vi "LVClass_Camera get all camera parameter values.vi"(0 "Camera in":refnum<class "Camera.lvclass">, 11 "error in (no error)":errorcluster) -> (4 "Camera out":refnum<class "Camera.lvclass">, 6 "ListOfSettableAndGettableValue":T1[](array[typedef]), 8 "nb_image":u32, 10 "BG Image OUT":refnum<class "Image.lvclass">, 15 "error out":errorcluster)   [LabVIEW 2020, in "Camera.lvclass"]
uses:
  Camera.lvclass
  Controls/CameraParametersSetup.ctl
  Controls/CameraParameters_Type.ctl
  Image/Image.lvclass
  Camera.lvclass/Camera.ctl
  LVClass_Camera Read acquisition state.vi
  LVClass_Camera Read all camera parameters.vi
  Image/LVClass_Image read Image Compat ptr.vi
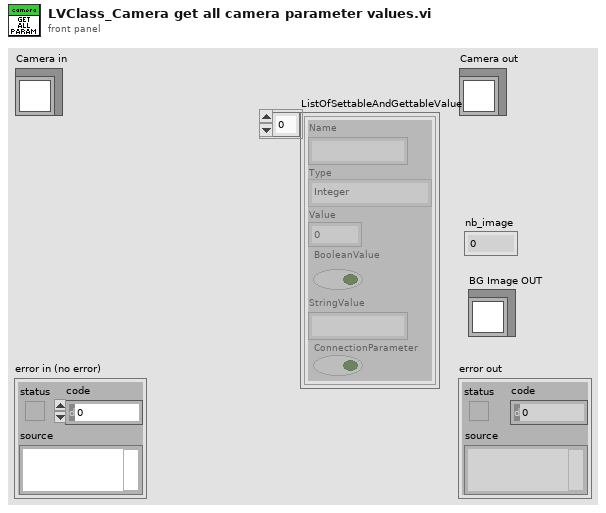
[diagram p1: front panel]
types:
  T1 = typedef "CameraParametersSetup.ctl" = cluster{"Name":string, "Type":T2, "Value":dbl, "BooleanValue":bool, "StringValue":string, "ConnectionParameter":bool}
  T2 = typedef "CameraParameters_Type.ctl" = enum16{"Integer", "Real", "String", "Boolean"}
  T3 = typedef "CameraAcquisitionState.ctl" = enum16{"Stop", "Live"}
  T4 = typedef "ParameterID.ctl" = cluster{"Name":string, "ConnectionParameter?":bool, "Type":T2, "Authorization":T5, "OnFlyAuthorization":T6, "StringValue":string, "Value":dbl, "Min":dbl, "Max":dbl, "BooleanValue":bool, "StringParameterList":string[]}
  T5 = typedef "CameraParameters_Authorization.ctl" = enum16{"Disable", "Gettable", "Settable - Gettable"}
  T6 = typedef "CameraParameters_OnFlyAuthorization.ctl" = enum16{"None", "Gettable", "Settable", "Settable - Gettable"}
  T7 = enum32{"invalid app kind", "Development System", "Run Time System", "Student Edition", "Embedded LabVIEW", "Evaluation", "Custom"}
  T8 = typedef "ClassID.ctl" = i64
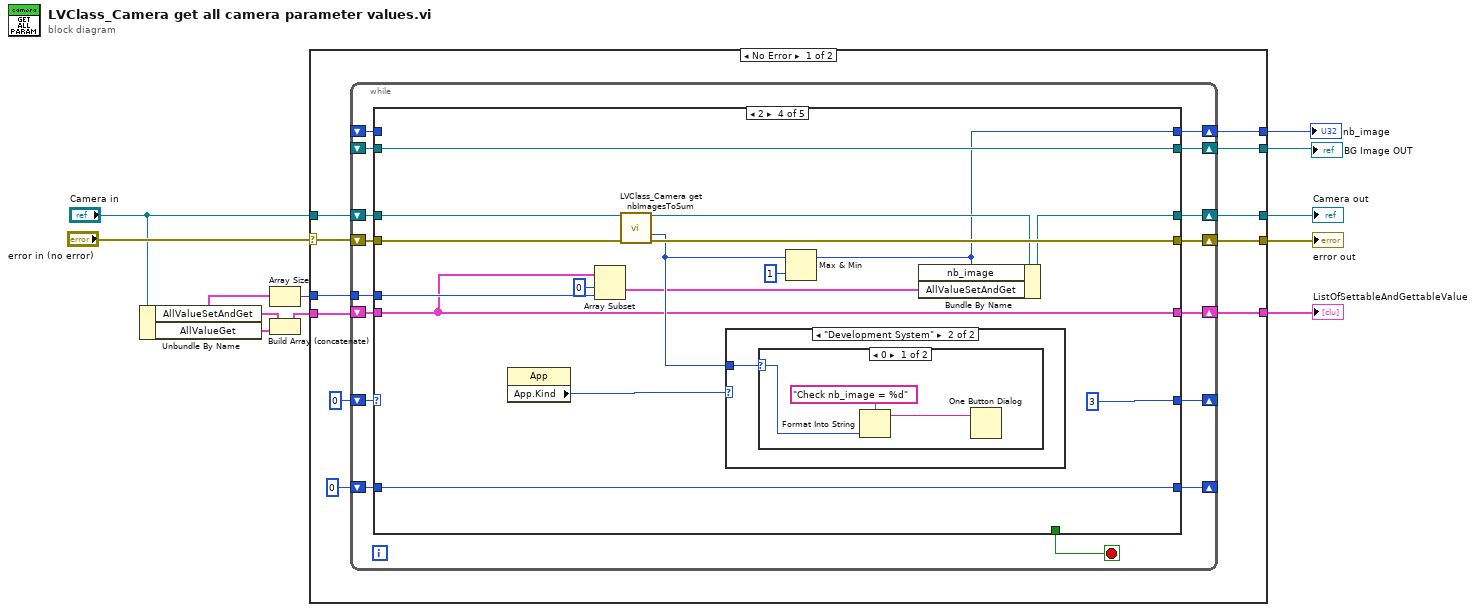
[diagram p0: block diagram]
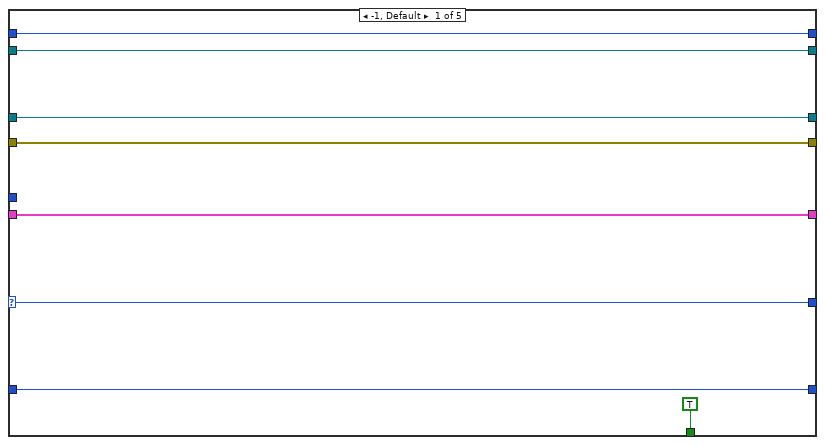
[diagram p2: hidden frame]
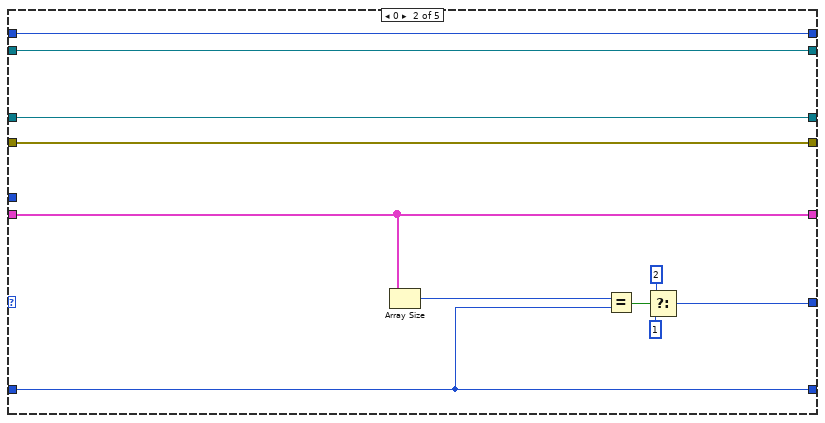
[diagram p3: hidden frame]
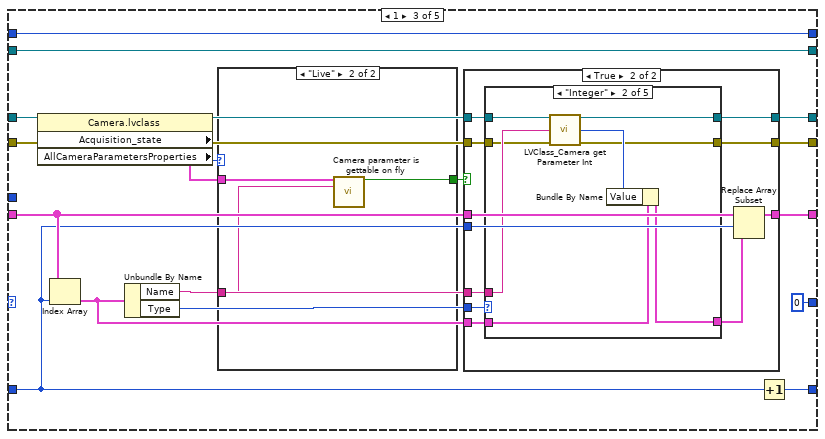
[diagram p4: hidden frame]
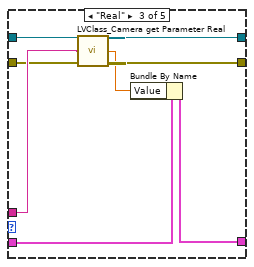
[diagram p7: hidden frame]
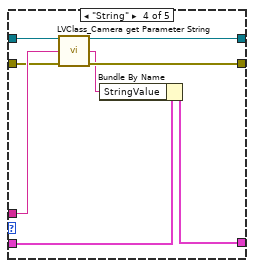
[diagram p8: hidden frame]
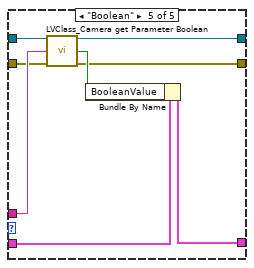
[diagram p9: hidden frame]
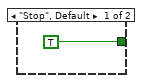
[diagram p10: hidden frame]
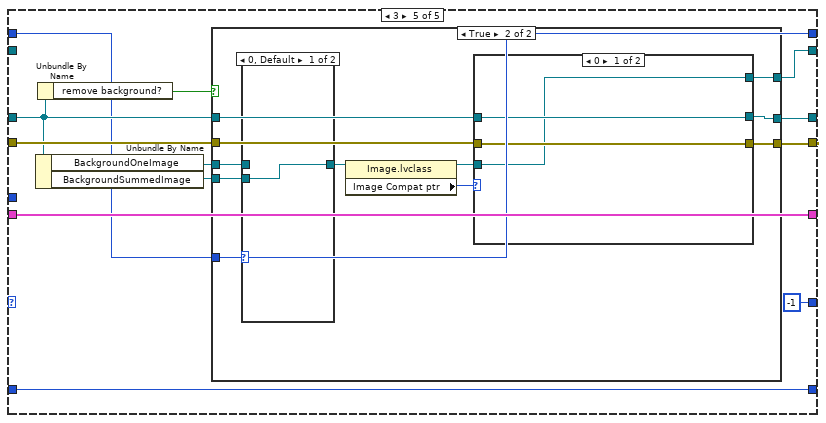
[diagram p13: hidden frame]
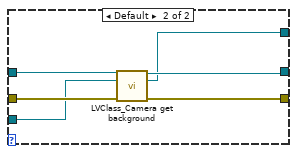
[diagram p16: hidden frame]
diagram:
  n1 = Unbundle By Name("Camera in") -> ("AllValueSetAndGet"=w1:T1[], "AllValueGet"=w4:T1[])
  n2 = Array Size(array=w1) -> (size(s)=w2:i32)
  n3 = Build Array (concatenate)(w1, w4) -> (w3:T1[])
  n4 = case shown="No Error" "error in (no error)" {
    selector: "error in (no error)" -> [w18 w188]
    tunnel: [w19 w188] -> w10
    tunnel: [w20 w187] -> w9
    tunnel: "Camera in" -> [w22 w187]
    tunnel: [w17 _] -> w8
    tunnel: [w16 _] -> w7
    tunnel: [w15 _] -> w6
    tunnel: w3 -> [w13 _]
    tunnel: w2 -> [w12 _]
    frame No Error {
      n5 = while {
        shift-right: [w37] -> _
        shift-left: 0 -> [w36]
        shift-right: [w34] -> w19
        shift-left: w18 -> [w33]
        shift-right: [w35] -> w20
        shift-left: w22 -> [w38]
        shift-right: [w30] -> w17
        shift-left: _ -> [w31]
        shift-right: [w29] -> w16
        shift-left: w13 -> [w28]
        shift-right: [w27] -> w15
        shift-left: _ -> [w26]
        shift-right: [w24] -> _
        shift-left: 0 -> [w25]
        tunnel: w12 -> [w23]
        stop <- w32 stop-if-true
        n6 = case shown="2" w36 {
          selector: w36 -> [w39 _ _ _ _]
          tunnel: w38 -> [w45 w57 w65 w144 w155]
          tunnel: w33 -> [w44 w56 w63 w143 w161]
          tunnel: [w39 w48 0 3 -1] -> w37
          tunnel: [w45 w57 w75 w139 w160] -> w35
          tunnel: [w44 w56 w74 w142 w159] -> w34
          tunnel: [TRUE _ _ _ _] -> w32
          tunnel: w31 -> [w43 w55 w73 w141 _]
          tunnel: [w43 w55 w73 w141 w158] -> w30
          tunnel: [w41 w53 w67 w132 w157] -> w29
          tunnel: w28 -> [w41 w53 w69 w132 w157]
          tunnel: [w42 w54 w72 w136 w152] -> w27
          tunnel: w26 -> [w42 w54 w72 _ w152]
          tunnel: w25 -> [w40 w51 w68 w138 w150]
          tunnel: [w40 w51 w71 w138 w150] -> w24
          tunnel: w23 -> [_ _ _ w133 _]
          frame -1, Default {
          }
          frame 0 {
            n7 = Array Size(array=w53) -> (size(s)=w52:i32)
            n8 = Equal?(x=w52, y=w51) -> (x = y?=w50:bool)
            n9 = Select(t=2, s=w50, f=1) -> (s? t:f=w48:i32)
          }
          frame 1 {
            n10 = property class="Camera.lvclass"(reference=w65, error in=w63) -> (reference out=w64:refnum<class "Camera.lvclass">, error out=w62:errorcluster, "Acquisition_state"=w61:T3, "AllCameraParametersProperties"=w60:T4[])
            n11 = Index Array(array=w69, index=w68) -> (element=w70:T1)
            n12 = Unbundle By Name(w70) -> ("Name"=w58:string, "Type"=w66:T2)
            n13 = case shown="\"Live\"" w61 {
              tunnel: w60 -> [_ w128]
              tunnel: [TRUE w129] -> w59
              tunnel: w58 -> [_ w127]
              frame "Stop", Default {
              }
              frame "Live" {
                n14 = call "Camera parameter is gettable on fly.vi"("AllCameraParameters"=w128, "Name"=w127) -> ("Gettable?"=w129:bool)  [unwired: 13 in]
              }
            }
            n15 = case shown="True" w59 {
              tunnel: [w79 w90] -> w75
              tunnel: [w78 w89] -> w74
              tunnel: w70 -> [_ w88]
              tunnel: w69 -> [w77 w87]
              tunnel: w68 -> [_ w86]
              tunnel: [w77 w85] -> w67
              tunnel: w66 -> [_ w84]
              tunnel: w58 -> [_ w83]
              tunnel: w64 -> [w79 w82]
              tunnel: w62 -> [w78 w81]
              frame False {
              }
              frame True {
                n16 = case shown="\"Integer\"" w84 {
                  tunnel: w88 -> [w91 w101 w102 w110 w119]
                  tunnel: [w91 w100 w103 w117 w118] -> w80
                  tunnel: w83 -> [_ w99 w108 w114 w124]
                  tunnel: w82 -> [w93 w98 w109 w116 w125]
                  tunnel: [w93 w97 w105 w115 w122] -> w90
                  tunnel: [w92 w95 w106 w112 w120] -> w89
                  tunnel: w81 -> [w92 w94 w107 w113 w123]
                  frame Default {
                  }
                  frame "Integer" {
                    n17 = call "LVClass_Camera get Parameter Int.vi"("Camera in"=w98, "parameter_name"=w99, "error in (no error)"=w94) -> ("Camera out"=w97:refnum<class "Camera.lvclass">, "value"=w96:i32, "error out"=w95:errorcluster)  [unwired: 10 in]
                    n18 = Bundle By Name(cluster=w101, "Value"=w96) -> (w100:T1)
                  }
                  frame "Real" {
                    n19 = call "LVClass_Camera get Parameter Real.vi"("Camera in"=w109, "parameter_name"=w108, "error in (no error)"=w107) -> ("Camera out"=w105:refnum<class "Camera.lvclass">, "value"=w104:dbl, "error out"=w106:errorcluster)  [unwired: 10 in]
                    n20 = Bundle By Name(cluster=w102, "Value"=w104) -> (w103:T1)
                  }
                  frame "String" {
                    n21 = call "LVClass_Camera get Parameter String.vi"("Camera in"=w116, "parameter_name"=w114, "error in (no error)"=w113) -> ("Camera out"=w115:refnum<class "Camera.lvclass">, "value"=w111:string, "error out"=w112:errorcluster)  [unwired: 10 in]
                    n22 = Bundle By Name(cluster=w110, "StringValue"=w111) -> (w117:T1)
                  }
                  frame "Boolean" {
                    n23 = call "LVClass_Camera get Parameter Boolean.vi"("Camera in"=w125, "parameter_name"=w124, "error in (no error)"=w123) -> ("Camera out"=w122:refnum<class "Camera.lvclass">, "value"=w121:bool, "error out"=w120:errorcluster)  [unwired: 10 in]
                    n24 = Bundle By Name(cluster=w119, "BooleanValue"=w121) -> (w118:T1)
                  }
                }
                n25 = Replace Array Subset(array=w87, new element=w80, index=w86) -> (w85:T1[])
              }
            }
            n26 = Increment(x=w68) -> (x+1=w71:i32)
          }
          frame 2 {
            n27 = property class="App"() -> ("App.Kind"=w135:T7)  [unwired: 2 in, 2 out]
            n28 = Array Subset(array=w132, index=0, length=w133) -> (w131:T1[])
            n29 = call "LVClass_Camera get nbImagesToSum.vi"("Camera in"=w144, "error in (no error)"=w143) -> ("Camera out"=w140:refnum<class "Camera.lvclass">, "nb_image"=w134:u32, "error out"=w142:errorcluster)  [unwired: 11 in]
            n30 = case shown="\"Development System\"" w135 {
              tunnel: w134 -> [_ w146]
              frame "invalid app kind", Default {
              }
              frame "Development System" {
                n31 = case shown="0" w146 {
                  selector: w146 -> [w149 _]
                  frame 0 {
                    n32 = Format Into String(format string="Check nb_image = %d" ("message"), w149) -> (resulting string=w147:string)  [unwired: 2 in, 1 out]
                    n33 = One Button Dialog(message=w147) -> ()  [unwired: 1 in, 1 out]
                  }
                  frame 1, Default {
                  }
                }
              }
            }
            n34 = Max & Min(x=w134, y=u32 1) -> (max(x,y)=w136:u32)  [unwired: 1 out]
            n35 = Bundle By Name(cluster=w140, "nb_image"=w136, "AllValueSetAndGet"=w131) -> (w139:refnum<class "Camera.lvclass">)
          }
          frame 3 {
            n36 = Unbundle By Name(w155) -> ("BackgroundOneImage"=w156:refnum<class "Image.lvclass">, "BackgroundSummedImage"=w151:refnum<class "Image.lvclass">)
            n37 = Unbundle By Name(w155) -> ("remove background?"=w153:bool)
            n38 = case shown="True" w153 {
              tunnel: w161 -> [w162 w174]
              tunnel: [w163 w173] -> w160
              tunnel: [w162 w172] -> w159
              tunnel: [w164 w171] -> w158
              tunnel: w156 -> [w164 w167]
              tunnel: w155 -> [w163 w170]
              tunnel: w152 -> [_ w168]
              tunnel: w151 -> [_ w165]
              frame False {
              }
              frame True {
                n39 = case shown="0, Default" w168 {
                  tunnel: w167 -> [_ w177]
                  tunnel: [w176 w177] -> w166
                  tunnel: w165 -> [w176 _]
                  frame 0, Default {
                  }
                  frame 1 {
                  }
                }
                n40 = property class="Image.lvclass"(reference=w166) -> (reference out=w169:refnum<class "Image.lvclass">, "Image Compat ptr"=w175:T8)  [unwired: 1 in, 1 out]
                n41 = case shown="0" w175 {
                  tunnel: w170 -> [w179 w186]
                  tunnel: w174 -> [w180 w185]
                  tunnel: [w179 w184] -> w173
                  tunnel: [w180 w183] -> w172
                  tunnel: [w178 w182] -> w171
                  tunnel: w169 -> [w178 w181]
                  frame 0 {
                  }
                  frame Default {
                    n42 = call "LVClass_Camera get background.vi"("Camera in"=w186, "BG Image IN"=w181, "error in (no error)"=w185) -> ("Camera out"=w184:refnum<class "Camera.lvclass">, "BG Image OUT"=w182:refnum<class "Image.lvclass">, "error out"=w183:errorcluster)  [unwired: 10 in]
                  }
                }
              }
            }
          }
        }
      }
    }
    frame Error {
    }
  }
  "error out" <- w10
  "Camera out" <- w9
  "ListOfSettableAndGettableValue" <- w7
  "nb_image" <- w6
  "BG Image OUT" <- w8
